vi "CMN_Efficiency.vi"(7 "Action":enum16{"ADD", "CLEAR", "GET", "GET LAST"}(ring), 9 "exptime":dbl format="%.2f", 10 "UTSHUT":string, 11 "size":u8=10) -> (2 "efficency":dbl format="%.4f")   [LabVIEW 2016]
panel:
  out "accum exp time":dbl format="%.2f"
  in  "point":cluster{"UTSHUT":dbl, "exptime":dbl} {"exptime" format="%.2f"; "UTSHUT" format="%.2f"}
  out "PointsArr":cluster{"UTSHUT":dbl, "exptime":dbl}[](array[cluster]) {"exptime" format="%.2f"; "UTSHUT" format="%.2f"}
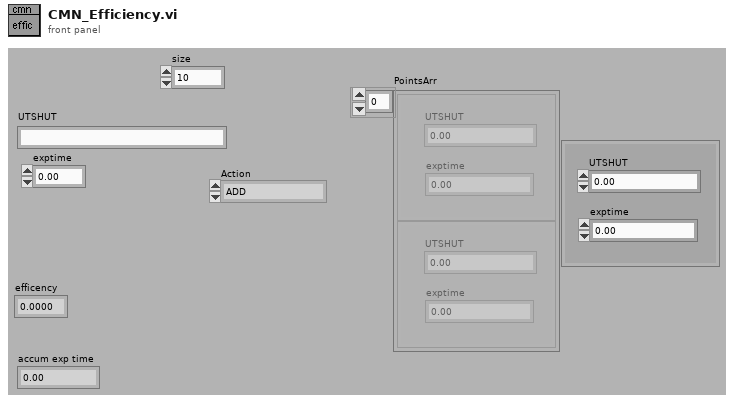
[diagram p1: front panel]
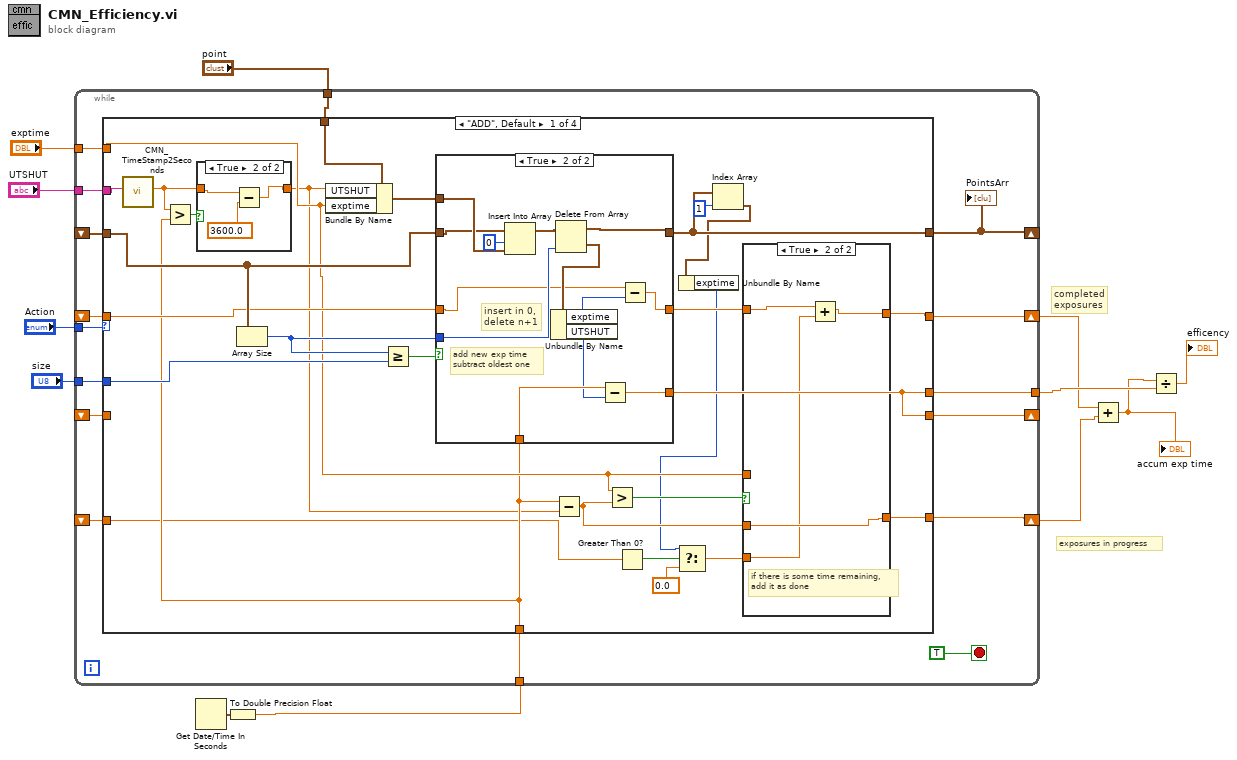
[diagram p0: block diagram]
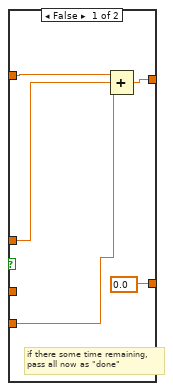
[diagram p3: hidden frame]
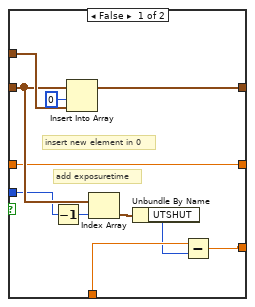
[diagram p4: hidden frame]
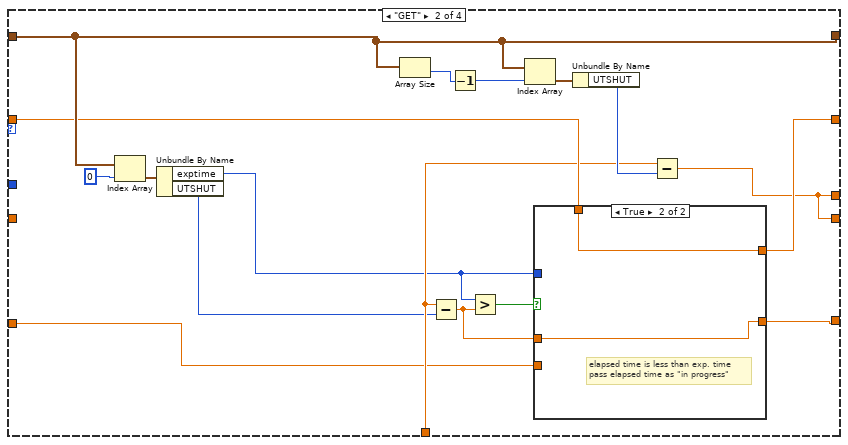
[diagram p5: hidden frame]
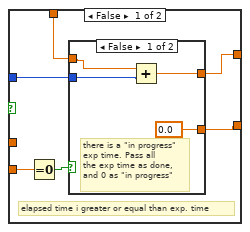
[diagram p6: hidden frame]
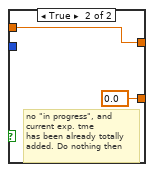
[diagram p7: hidden frame]
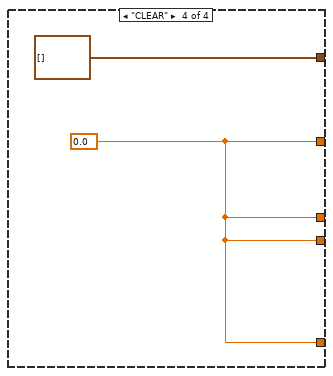
[diagram p9: hidden frame]
diagram:
  # "exposures in progress"
  # "completed \nexposures"
  n1 = Get Date/Time In Seconds() -> (seconds since 1Jan1904=w1:timestamp)
  n2 = To Double Precision Float(number=w1) -> (double precision float=w5:dbl)
  n3 = while {
    tunnel: "Action" -> [w27]
    tunnel: "exptime" -> [w26]
    tunnel: "UTSHUT" -> [w25]
    tunnel: "point" -> [w24]
    tunnel: "size" -> [w23]
    shift-right: [w21] -> _
    shift-left: _ -> [w22]
    shift-right: [w20] -> w4
    shift-left: _ -> [w19]
    tunnel: w5 -> [w18]
    tunnel: [w17] -> w7
    shift-right: [w16] -> w3
    shift-left: _ -> [w15]
    shift-right: [w14] -> _
    shift-left: _ -> [w13]
    stop <- TRUE stop-if-true
    n4 = case shown="\"ADD\", Default" w27 {
      tunnel: w26 -> [w42 _ _ _]
      tunnel: w25 -> [w55 _ _ _]
      tunnel: w24 -> [w54 _ _ _]
      tunnel: w23 -> [w51 _ _ _]
      tunnel: [w36 w105 w124 cluster{"UTSHUT":u32, "exptime":u32}[] []] -> w21
      tunnel: w22 -> [w50 w105 w124 _]
      tunnel: [w44 w95 w127 w128] -> w20
      tunnel: w19 -> [w46 w102 w127 _]
      tunnel: w18 -> [w41 w101 _ _]
      tunnel: [w37 w93 w125 w128] -> w17
      tunnel: [w43 w96 w126 w128] -> w16
      tunnel: w15 -> [w34 w94 w126 _]
      tunnel: [w37 w93 w125 w128] -> w14
      tunnel: w13 -> [_ _ w125 _]
      frame "ADD", Default {
        n5 = call "CMN_TimeStamp2Seconds.vi"("TimeStamp string (yyyy-mm-ddThh:mm:ss)"=w55) -> ("seconds out"=w39:dbl)  [unwired: 1 in, 8 out]
        n6 = Greater?(x=w39, y=w41) -> (0:w40:bool)
        n7 = case shown="True" w40 {
          tunnel: w39 -> [w56 w59]
          tunnel: [w56 w57] -> w38
          frame False {
          }
          frame True {
            n8 = Subtract(x=w59, y=3600.0) -> (x-y=w57:dbl)
          }
        }
        n9 = Array Size(array=w50) -> (size(s)=w49:i32)
        n10 = Bundle By Name(cluster=w54, "UTSHUT"=w38, "exptime"=w42) -> (w53:cluster{"UTSHUT":dbl, "exptime":dbl})
        n11 = Greater Or Equal?(x=w49, y=w51) -> (x >= y?=w52:bool)
        n12 = case shown="True" w52 {
          tunnel: w53 -> [w79 w91]
          tunnel: [w77 w88] -> w36
          tunnel: w50 -> [w76 w90]
          tunnel: w49 -> [w75 w87]
          tunnel: w41 -> [w72 w84]
          tunnel: [w70 w82] -> w37
          tunnel: w46 -> [w69 w80]
          tunnel: [w69 w81] -> w45
          frame False {
            # "add exposuretime"
            # "insert new element in 0"
            n13 = Decrement(x=w75) -> (x-1=w74:i32)
            n14 = Insert Into Array(array=w76, index=0, new element=w79) -> (w77:cluster{"UTSHUT":u32, "exptime":u32}[])
            n15 = Index Array(array=w76, index=w74) -> (element=w73:cluster{"UTSHUT":u32, "exptime":u32})
            n16 = Unbundle By Name(w73) -> ("UTSHUT"=w71:u32)
            n17 = Subtract(x=w72, y=w71) -> (x-y=w70:dbl)
          }
          frame True {
            # "add new exp time\nsubtract oldest one"
            # "insert in 0,\ndelete n+1"
            n18 = Insert Into Array(array=w90, index=0, new element=w91) -> (w89:cluster{"UTSHUT":u32, "exptime":u32}[])
            n19 = Delete From Array(array=w89, index=w87) -> (deleted portion=w85:cluster{"UTSHUT":u32, "exptime":u32}, array with subset deleted=w88:cluster{"UTSHUT":u32, "exptime":u32}[])  [unwired: 1 in]
            n20 = Unbundle By Name(w85) -> ("exptime"=w86:u32, "UTSHUT"=w83:u32)
            n21 = Subtract(x=w84, y=w83) -> (x-y=w82:dbl)
            n22 = Subtract(x=w80, y=w86) -> (x-y=w81:dbl)
          }
        }
        n23 = Subtract(x=w41, y=w38) -> (x-y=w48:dbl)
        n24 = Greater?(x=w42, y=w48) -> (0:w47:bool)
        n25 = Greater Than 0?(x=w34) -> (x > 0?=w33:bool)
        n26 = Index Array(array=w36, index=1) -> (element=w31:cluster{"UTSHUT":u32, "exptime":u32})
        n27 = Unbundle By Name(w31) -> ("exptime"=w30:u32)
        n28 = Select(t=w30, s=w33, f=0.0) -> (s? t:f=w29:dbl)
        n29 = case shown="True" w47 {
          tunnel: w42 -> [w63 _]
          tunnel: w48 -> [_ w68]
          tunnel: w45 -> [w64 w67]
          tunnel: [w61 w65] -> w44
          tunnel: [0.0 w68] -> w43
          tunnel: w29 -> [w60 w66]
          frame False {
            # "if there some time remaining,\npass all now as \"done\""
            n30 = Compound Arithmetic op=ADD(w64, w63, w60) -> (w61:dbl)
          }
          frame True {
            # "if there is some time remaining,\nadd it as done"
            n31 = Add(x=w67, y=w66) -> (x+y=w65:dbl)
          }
        }
      }
      frame "GET" {
        n32 = Index Array(array=w105, index=0) -> (element=w103:cluster{"UTSHUT":u32, "exptime":u32})
        n33 = Unbundle By Name(w103) -> ("exptime"=w99:u32, "UTSHUT"=w100:u32)
        n34 = Array Size(array=w105) -> (size(s)=w109:i32)
        n35 = Subtract(x=w101, y=w100) -> (x-y=w97:dbl)
        n36 = Decrement(x=w109) -> (x-1=w108:i32)
        n37 = Greater?(x=w99, y=w97) -> (0:w98:bool)
        n38 = Index Array(array=w105, index=w108) -> (element=w107:cluster{"UTSHUT":u32, "exptime":u32})
        n39 = case shown="True" w98 {
          tunnel: w102 -> [w112 w122]
          tunnel: w99 -> [w111 _]
          tunnel: w97 -> [_ w123]
          tunnel: [w113 w123] -> w96
          tunnel: [w110 w122] -> w95
          tunnel: w94 -> [w114 _]
          frame False {
            # "elapsed time i greater or equal than exp. time"
            n40 = Equal To 0?(x=w114) -> (x = 0?=w115:bool)
            n41 = case shown="False" w115 {
              tunnel: [0.0 0.0] -> w113
              tunnel: w112 -> [w118 w121]
              tunnel: w111 -> [w117 _]
              tunnel: [w116 w121] -> w110
              frame False {
                # "there is a \"in progress\"\nexp time. Pass all\nthe exp time as done,\nand 0 as \"in progress\""
                n42 = Add(x=w118, y=w117) -> (x+y=w116:dbl)
              }
              frame True {
                # "no \"in progress\", and\ncurrent exp. tme\nhas been already totally\nadded. Do nothing then"
              }
            }
          }
          frame True {
            # "elapsed time is less than exp. time\npass elapsed time as \"in progress\""
          }
        }
        n43 = Unbundle By Name(w107) -> ("UTSHUT"=w106:u32)
        n44 = Subtract(x=w101, y=w106) -> (x-y=w93:dbl)
      }
      frame "GET LAST" {
      }
      frame "CLEAR" {
        w128 = 0.0
      }
    }
    "PointsArr" <- w21
  }
  n45 = Add(x=w4, y=w3) -> (x+y=w2:dbl)
  "accum exp time" <- w2
  n46 = Divide(x=w2, y=w7) -> (x/y=→"efficency":dbl)
